vi "at.vi"(10 "\"At\" location":T1, 11 "String in":string) -> (3 "String out":string)   [LabVIEW 2013]
uses:
  at.ctl
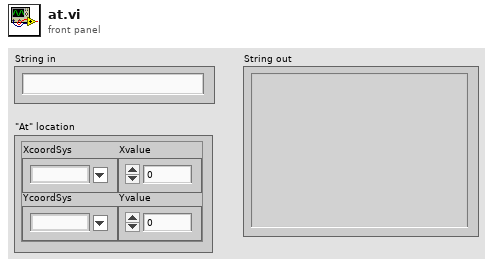
[diagram p1: front panel]
types:
  T1 = typedef "at.ctl" = cluster{"XcoordSys":string, "YcoordSys":string, "Xvalue":dbl, "Yvalue":dbl}
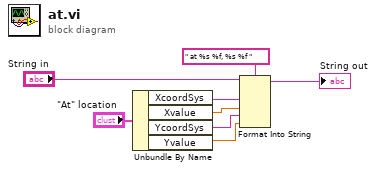
[diagram p0: block diagram]
diagram:
  n1 = Unbundle By Name("\"At\" location") -> ("XcoordSys"=w5:string, "Xvalue"=w4:dbl, "YcoordSys"=w3:string, "Yvalue"=w2:dbl)
  n2 = Format Into String(format string=" at %s %f, %s %f ", initial string="String in", w5, w4, w3, w2) -> (resulting string=→"String out":string)  [unwired: 1 in, 1 out]
